vi "Do Rename Object.vi"(8 "error in (no error)":errorcluster, 10 "rename_object Argument":T2, 11 "Data Cluster in":T1) -> (0 "error out":errorcluster, 3 "Data Cluster out":T1)   [LabVIEW 2025, in "Scripting Server.lvlib"]
uses:
  Scripting Server.lvlib
  rename_object (Reply Payload)--cluster.ctl
  rename_object Argument--cluster.ctl
  Module Data--cluster.ctl
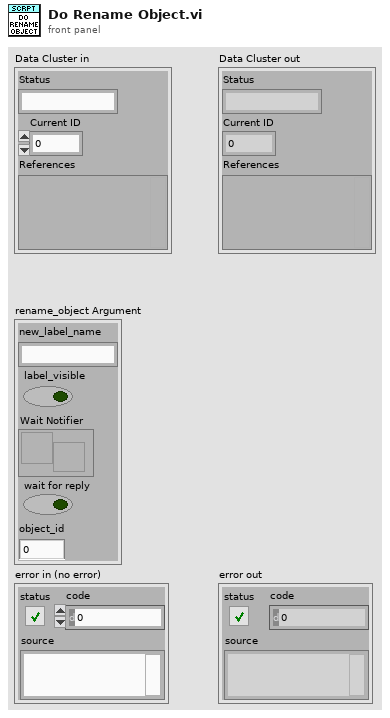
[diagram p1: front panel]
types:
  T1 = typedef "Scripting Server.lvlib/Module Data--cluster.ctl" = cluster{"Status":string, "Current ID":i32, "References":variant}
  T2 = typedef "Scripting Server.lvlib/rename_object Argument--cluster.ctl" = cluster{"new_label_name":string, "label_visible":bool, "Wait Notifier":refnum<notifier>, "wait for reply":bool, "object_id":i32}
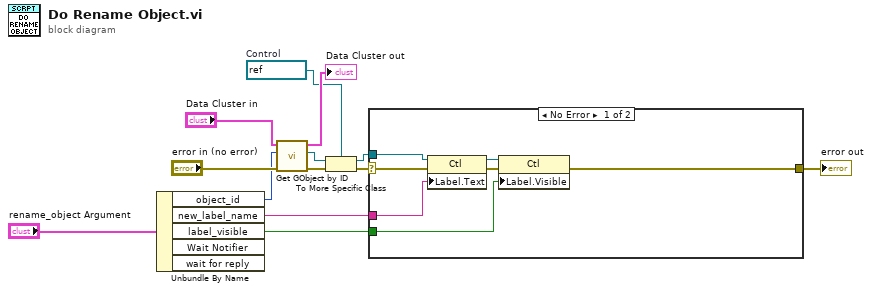
[diagram p0: block diagram]
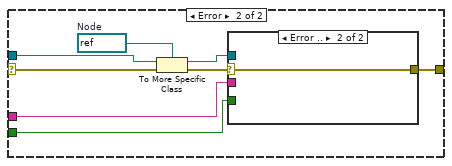
[diagram p2: hidden frame]
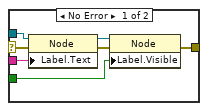
[diagram p3: hidden frame]
diagram:
  w5 = refnum<vi> refnum  # Control
  n1 = Unbundle By Name("rename_object Argument") -> ("object_id"=w8:i32, "new_label_name"=w4:string, "label_visible"=w2:bool)  [unwired: 2 out]
  n2 = call "Get GObject by ID.vi"("error in (no error)"="error in (no error)", "ID"=w8, "Data Cluster in"="Data Cluster in") -> ("error out"=w11:errorcluster, "gobject"=w7:refnum<vi>, "Data Cluster out"=→"Data Cluster out":T1)  [unwired: 6 in]
  n3 = To More Specific Class(target class=w5, reference=w7, error in=w11) -> (specific class reference=w6:refnum<vi>, error out=w3:errorcluster)
  n4 = case shown="No Error" w3 {
    selector: w3 -> [w18 w28]
    tunnel: w6 -> [w20 w27]
    tunnel: w4 -> [w19 w21]
    tunnel: w2 -> [w16 w22]
    tunnel: [w15 w25] -> w1
    frame No Error {
      n5 = property class="Ctl"(reference=w20, error in=w18, "Label.Text"=w19) -> (reference out=w17:refnum<vi>, error out=w14:errorcluster)
      n6 = property class="Ctl"(reference=w17, error in=w14, "Label.Visible"=w16) -> (error out=w15:errorcluster)  [unwired: 1 out]
    }
    frame Error {
      w26 = refnum<vi> refnum  # Node
      n7 = To More Specific Class(target class=w26, reference=w27, error in=w28) -> (specific class reference=w23:refnum<vi>, error out=w24:errorcluster)
      n8 = case shown="Error .." w24 {
        selector: w24 -> [w34 w36]
        tunnel: [w32 w36] -> w25
        tunnel: w23 -> [w33 _]
        tunnel: w22 -> [w30 _]
        tunnel: w21 -> [w29 _]
        frame No Error {
          n9 = property class="Node"(reference=w33, error in=w34, "Label.Text"=w29) -> (reference out=w31:refnum<vi>, error out=w35:errorcluster)
          n10 = property class="Node"(reference=w31, error in=w35, "Label.Visible"=w30) -> (error out=w32:errorcluster)  [unwired: 1 out]
        }
        frame Error {
        }
      }
    }
  }
  "error out" <- w1
